vi "Read ALR_index.vi"(11 "valve_VCH in":refnum<class "valve_VCH.lvclass">) -> (2 "ALR_index":i32[](array[numeric]), 3 "valve_VCH out":refnum<class "valve_VCH.lvclass">)   [LabVIEW 2019, in "valve_VCH.lvclass"]
uses:
  valve_VCH.lvclass
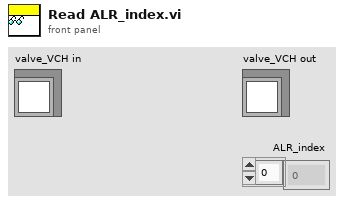
[diagram p1: front panel]
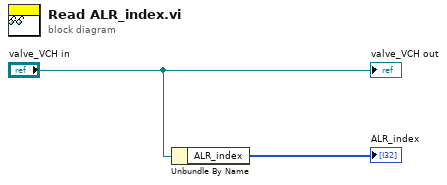
[diagram p0: block diagram]
diagram:
  n1 = Unbundle By Name("valve_VCH in") -> ("ALR_index"=→"ALR_index":i32[])
  "valve_VCH out" <- "valve_VCH in"
